vi "M04 Smart Grid.vi"(9 "Target angle":sgl, 11 "EV3 in":T1) -> (3 "EV3 out":T1)   [LabVIEW 2016]
uses:
  <vilib>/NXT/Subs/LVHSConnector.ctl
  <vilib>/NXT/LegoClasses/BrickReference/BrickReference.lvclass
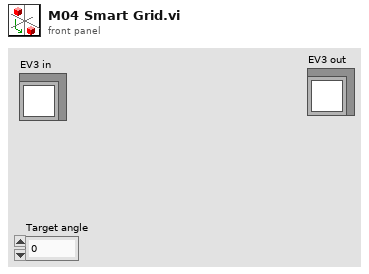
[diagram p1: front panel]
types:
  T1 = typedef "LVHSConnector.ctl" = refnum<class "BrickReference.lvclass">
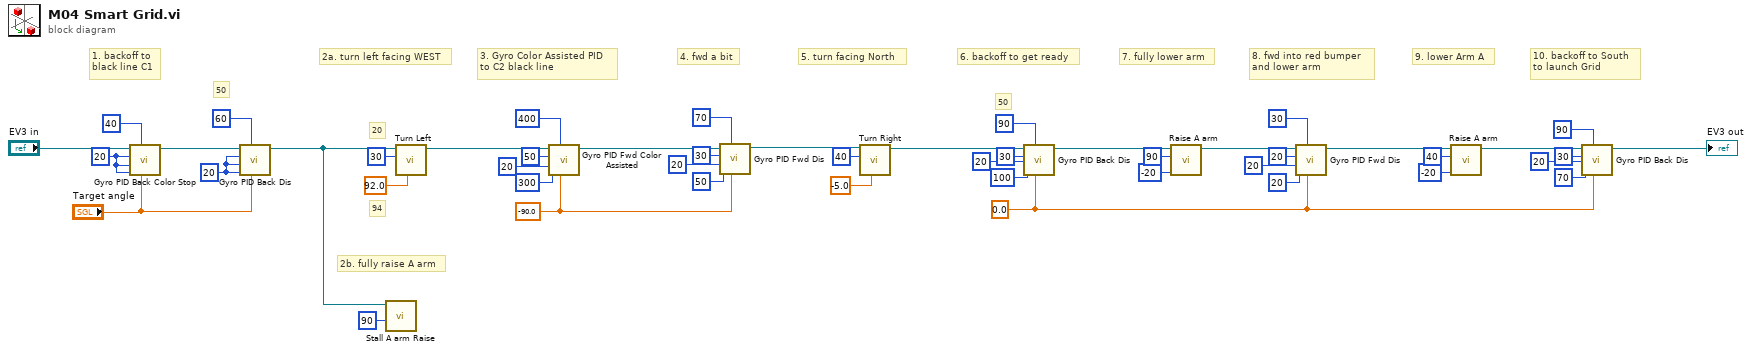
[diagram p0: block diagram]
diagram:
  w13 = 20 ("Max. speed")
  w2 = sgl 0.0 ("Target angle")
  w23 = 20 ("Max. speed")
  w37 = sgl -90.0 ("Target angle")
  # "9. lower Arm A"
  # "50"
  # "8. fwd into red bumper\nand lower arm"
  # "20"
  # "94"
  # "50"
  # "7. fully lower arm"
  # "6. backoff to get ready"
  # "2b. fully raise A arm"
  # "1. backoff to\nblack line C1"
  # "10. backoff to South\nto launch Grid"
  # "5. turn facing North"
  # "4. fwd a bit"
  # "3. Gyro Color Assisted PID\nto C2 black line"
  # "2a. turn left facing WEST"
  n1 = call "Gyro PID Back Color Stop.vi"("Target angle"="Target angle", "Threshold to Color"=40, "Threshold to slow"=w23, "Min. speed"=w23, "Max. speed"=w23, "EV3 in"="EV3 in") -> ("EV3 out"=w16:T1)  [unwired: 5 in]
  n2 = call "Gyro PID Back Dis.vi"("Target angle"="Target angle", "Threshold to stop"=60, "Threshold to slow"=w13, "Min. speed"=w13, "Max. speed"=w13, "EV3 in"=w16) -> ("EV3 out"=w15:T1)  [unwired: 5 in]
  n3 = call "Stall A arm Raise.vi"("Power"=i8 90, "NXT/EV3"=w15) -> ()  [unwired: 9 in, 1 out]
  n4 = call "Turn Left.vi"("Turning angle"=sgl 92.0, "Motor B (right)"=i8 30, "EV3 in"=w15) -> ("EV3 out"=w28:T1)  [unwired: 8 in]
  n5 = call "Gyro PID Fwd Color Assisted.vi"("Target angle"=w37, "Threshold to Color"=400, "Threshold to slow"=300, "Min. speed"=20, "Max. speed"=50, "EV3 in"=w28) -> ("EV3 out"=w42:T1)  [unwired: 5 in]
  n6 = call "Gyro PID Fwd Dis.vi"("Target angle"=w37, "Threshold to stop"=70, "Threshold to slow"=50, "Min. speed"=20, "Max. speed"=30, "EV3 in"=w42) -> ("EV3 out"=w36:T1)  [unwired: 5 in]
  n7 = call "Turn Right.vi"("Turning angle"=sgl -5.0, "Motor B (right)"=i8 40, "EV3 in"=w36) -> ("EV3 out"=w18:T1)  [unwired: 8 in]
  n8 = call "Gyro PID Back Dis.vi"("Target angle"=w2, "Threshold to stop"=90, "Threshold to slow"=100, "Min. speed"=20, "Max. speed"=30, "EV3 in"=w18) -> ("EV3 out"=w17:T1)  [unwired: 5 in]
  n9 = call "Raise A arm.vi"("Power"=i8 -20, "Rotation"=90, "EV3 in"=w17) -> ("EV3 out"=w7:T1)  [unwired: 8 in]
  n10 = call "Gyro PID Fwd Dis.vi"("Target angle"=w2, "Threshold to stop"=30, "Threshold to slow"=20, "Min. speed"=20, "Max. speed"=20, "EV3 in"=w7) -> ("EV3 out"=w6:T1)  [unwired: 5 in]
  n11 = call "Raise A arm.vi"("Power"=i8 -20, "Rotation"=40, "EV3 in"=w6) -> ("EV3 out"=w5:T1)  [unwired: 8 in]
  n12 = call "Gyro PID Back Dis.vi"("Target angle"=w2, "Threshold to stop"=90, "Threshold to slow"=70, "Min. speed"=20, "Max. speed"=30, "EV3 in"=w5) -> ("EV3 out"=→"EV3 out":T1)  [unwired: 5 in]
